vi "svl_Log View for Energy Level (Resampled Signal).vi"(7 "resampled channel info":T1={"channel name"="", "description"="", " channel info"={"sensor sensitivity"=1000.0, "engineering units"=1, "dB reference"=1.0, "custom label"="EU", "weighting filter"=0, "pregain"=0.0}} {"channel info"."pregain" format="%.2f"; "channel info"."weighting filter" items=["Linear", "A-weighting", "B-weighting", "C-weighting", "ITU-R 468-4", "Dolby", "CCITT", "C-message", "Wb", "Wc", "Wd", "We", "Wf", "Wh", "Wj", "Wk", "Wm", "AES17 20 kHz lowpass", "AES17 40 kHz lowpass", "AES17 20 kHz highpass", "AES17 40 kHz highpass"]; "channel info"."dB reference" format="%^.1e"; "channel info"."engineering units" items=["custom..."=0, "V"=1, "A"=21, "C"=30, "pC"=31, "s"=32, "-"=29, "Pa"=2, "N"=20, "g"=3, "m/s^2"=4, "m/s"=5, "m"=6, "mm/s"=12, "mm"=13, "micron/s"=14, "micron"=15, "in/s^2"=7, "in/s"=8, "in"=9, "mil/s"=10, "mil"=11, "rad/s^2"=16, "rad/s"=17, "rad"=18, "deg/s^2"=26, "deg/s"=27, "deg"=28, "RPM"=22, "cycle/s^2"=23, "Hz"=24, "cycle"=25, "strain"=19]; "channel info"."sensor sensitivity" format="%#_5f"}, 8 "error in (no error)":errorcluster, 9 "view mode":enum16{"Power", "Amplitude"}(ring), 10 "dB On (T)":bool=TRUE, 11 "even angle signal":T5 {"even angle signal" format="%.2f"; "dr" format="%.2f"; "r0" format="%.2f"}) -> (0 "error out":errorcluster, 2 "unit label":string, 3 "even angle signal":T5 {"even angle signal" format="%.2f"; "dr" format="%.2f"; "r0" format="%.2f"})   [LabVIEW 2017]
uses:
  <vilib>/addons/_NISVFA/_Shared subVIs/Controls/svc_Resampled Channel Info.ctl
  <vilib>/addons/_NISVFA/_Shared subVIs/Controls/svc_Channel Info.ctl
  <vilib>/addons/_NISVFA/_Shared subVIs/Controls/svc_Engineering Units Text Ring.ctl
  <vilib>/addons/_NISVFA/_Shared subVIs/Controls/svc_Weighting Filter Text Ring.ctl
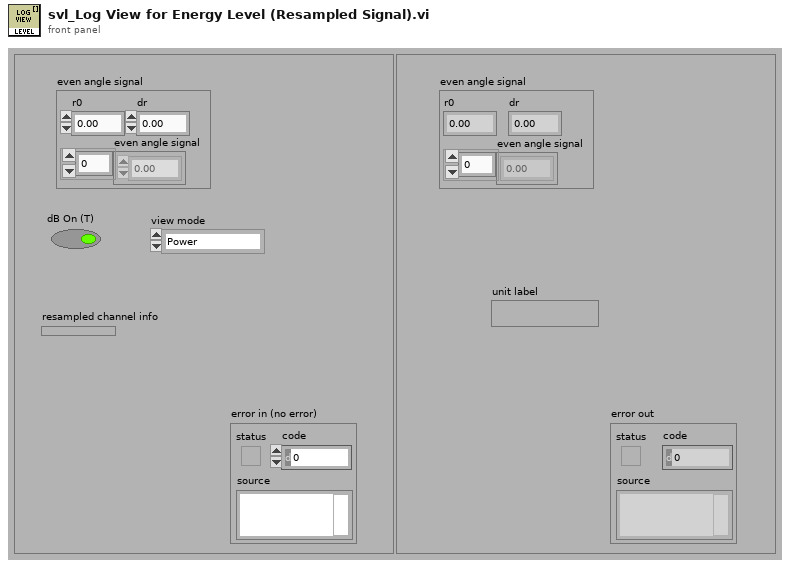
[diagram p1: front panel]
types:
  T1 = typedef "svc_Resampled Channel Info.ctl" = cluster{"channel name":string, "description":string, " channel info":T2}
  T2 = typedef "svc_Channel Info.ctl" = cluster{"sensor sensitivity":dbl, "engineering units":T3, "dB reference":dbl, "custom label":string, "weighting filter":T4, "pregain":dbl}
  T3 = typedef "svc_Engineering Units Text Ring.ctl" = u16
  T4 = typedef "svc_Weighting Filter Text Ring.ctl" = u16
  T5 = cluster{"r0":dbl, "dr":dbl, "even angle signal":dbl[]}
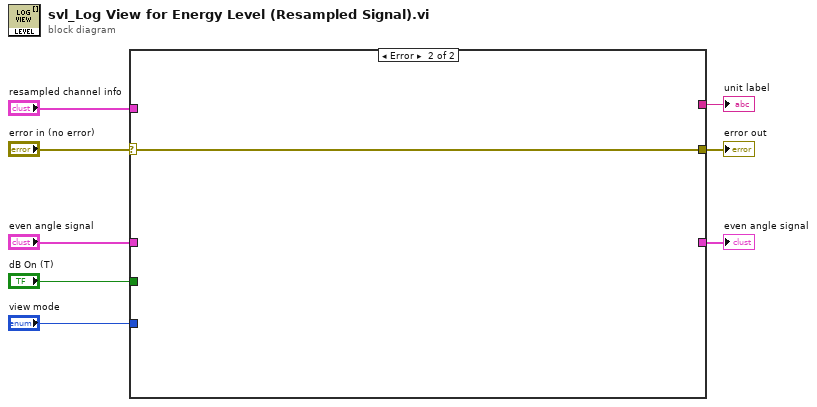
[diagram p0: block diagram]
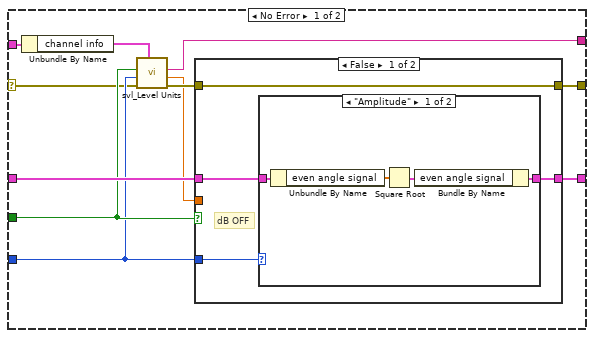
[diagram p2: hidden frame]
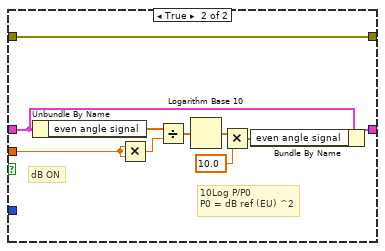
[diagram p4: hidden frame]
diagram:
  n1 = case shown="Error" "error in (no error)" {
    selector: "error in (no error)" -> [w9 w39]
    tunnel: [w19 w39] -> w8
    tunnel: "even angle signal" -> [w18 _]
    tunnel: [w17 _] -> w6
    tunnel: "dB On (T)" -> [w16 _]
    tunnel: "view mode" -> [w15 _]
    tunnel: [w12 _] -> w3
    tunnel: "resampled channel info" -> [w11 _]
    frame No Error {
      n2 = Unbundle By Name(w11) -> ("channel info"=w10:T2)
      n3 = call <vilib>:"svl_Level Units.vi"("channel info"=w10, "error in (no error)"=w9, "view mode"=w15, "dB On (T)"=w16) -> ("error out"=w14:errorcluster, "dB reference [EU]"=w13:dbl, "unit label"=w12:string)  [unwired: 5 in]
      n4 = case shown="False" w16 {
        tunnel: [w23 w29] -> w17
        tunnel: w14 -> [w22 w38]
        tunnel: [w22 w38] -> w19
        tunnel: w18 -> [w20 w30]
        tunnel: w15 -> [w21 _]
        tunnel: w13 -> [_ w33]
        frame False {
          # "dB OFF"
          n5 = case shown="\"Amplitude\"" w21 {
            tunnel: [w25 w28] -> w23
            tunnel: w20 -> [w26 w28]
            frame "Amplitude" {
              n6 = Unbundle By Name(w26) -> ("even angle signal"=w27:dbl[])
              n7 = Square Root(x=w27) -> (sqrt(x)=w24:dbl[])
              n8 = Bundle By Name(cluster=w26, "even angle signal"=w24) -> (w25:T5)
            }
            frame "Power", Default {
            }
          }
        }
        frame True {
          # "10Log P/P0\nP0 = dB ref (EU) ^2"
          # "dB ON"
          n9 = Unbundle By Name(w30) -> ("even angle signal"=w32:dbl[])
          n10 = Multiply(x=w33, y=w33) -> (x*y=w34:dbl)
          n11 = Divide(x=w32, y=w34) -> (x/y=w35:dbl[])
          n12 = Logarithm Base 10(1:w35) -> (0:w36:dbl[])
          n13 = Multiply(x=w36, y=10.0) -> (x*y=w31:dbl[])
          n14 = Bundle By Name(cluster=w30, "even angle signal"=w31) -> (w29:T5)
        }
      }
    }
    frame Error {
    }
  }
  "unit label" <- w3
  "even angle signal" <- w6
  "error out" <- w8
